vi "Taikoi_GetSystemStatus.vi"(8 "error in (no error)":errorcluster, 10 "LBSysStatRef":refnum<vi>, 11 "USBIdx":i32) -> (0 "error out":errorcluster, 1 "QError":bool, 2 "needUpdate":bool, 3 "Status":string)   [LabVIEW 2019]
uses:
  <userlib>/TaikoLaser/PDLM_Status.ctl
  <userlib>/TaikoLaser/PDLM_NamedBit.ctl
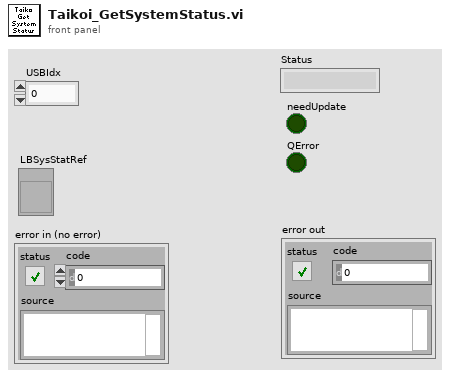
[diagram p1: front panel]
types:
  T1 = typedef "PDLM_Status.ctl" = T2[]
  T2 = typedef "PDLM_NamedBit.ctl" = cluster{"StatName":string, "StatBit":bool}
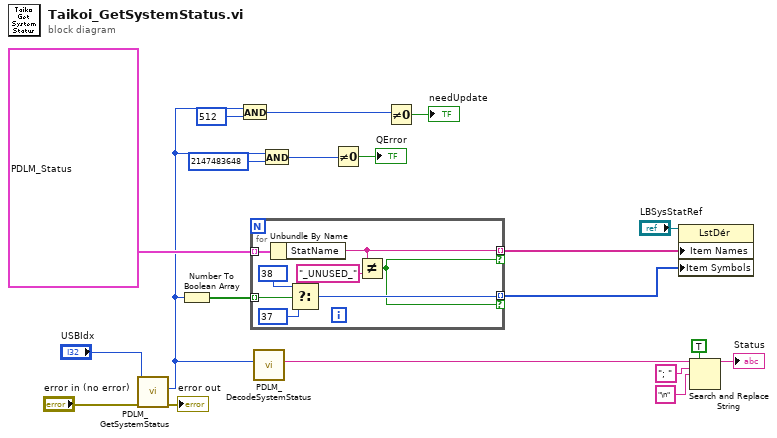
[diagram p0: block diagram]
diagram:
  n1 = call <userlib>:"PDLM_GetSystemStatus.vi"("error in (no error)"="error in (no error)", "USBIdx"="USBIdx") -> ("error out"=→"error out":errorcluster, "state"=w3:u32)  [unwired: 7 in, 1 out]
  n2 = Number To Boolean Array(number=w3) -> (Boolean array=w17:bool[])
  n3 = And(x=w3, y=u32 512) -> (x .and. y?=w6:u32)
  n4 = for {
    tunnel: w17 -> [w27] mode=indexing
    tunnel: T1 [{"StatName"="INITIALIZING", "StatBit"=FALSE}, {"StatName"="DEVICE_UNCALIBRATED", "StatBit"=FALSE}, {"StatName"="COMMISSIONING_MODE", "StatBit"=FALSE}, {"StatName"="LASERHEAD_SAFETY_MODE", "StatBit"=FALSE}, {"StatName"="FW_UPDATE_RUNNING", "StatBit"=FALSE}, {"StatName"="DEVICE_DEFECT", "StatBit"=FALSE}, {"StatName"="DEVICE_INCOMPATIBLE", "StatBit"=FALSE}, {"StatName"="BUSY", "StatBit"=FALSE}, {"StatName"="EXCLUSIVE_SW_OP_GRANTED", "StatBit"=FALSE}, {"StatName"="PARAMETER_CHANGES_PENDING", "StatBit"=FALSE}, {"StatName"="_UNUSED_", "StatBit"=FALSE}, {"StatName"="LASERHEAD_CHANGED", "StatBit"=FALSE}, {"StatName"="LASERHEAD_MISSING", "StatBit"=FALSE}, {"StatName"="LASERHEAD_DEFECT", "StatBit"=FALSE}, {"StatName"="LASERHEAD_UNKNOWN_TYPE", "StatBit"=FALSE}, {"StatName"="LASERHEAD_DECALIBRATED", "StatBit"=FALSE}, {"StatName"="LASERHEAD_DIODE_TEMP_TOO_LOW", "StatBit"=FALSE}, {"StatName"="LASERHEAD_DIODE_TEMP_TOO_HIGH", "StatBit"=FALSE}, {"StatName"="LASERHEAD_DIODE_OVERHEATING", "StatBit"=FALSE}, {"StatName"="LASERHEAD_CASE_OVERHEATING", "StatBit"=FALSE}, {"StatName"="LASERHEAD_FAN_RUNNING", "StatBit"=FALSE}, {"StatName"="LASERHEAD_INCOMPATIBLE", "StatBit"=FALSE}, {"StatName"="LOCKED_BY_EXPIRED_DEMO_MODE", "StatBit"=FALSE}, {"StatName"="LOCKED_BY_ON_OFF_BUTTON", "StatBit"=FALSE}, {"StatName"="SOFTLOCK", "StatBit"=FALSE}, {"StatName"="KEYLOCK", "StatBit"=FALSE}, {"StatName"="LOCKED_BY_SECURITY_POLICY", "StatBit"=FALSE}, {"StatName"="INTERLOCK", "StatBit"=FALSE}, {"StatName"="LASERHEAD_PULSE_POWER_INACCURATE", "StatBit"=FALSE}, {"StatName"="_UNUSED_", "StatBit"=FALSE}, {"StatName"="_UNUSED_", "StatBit"=FALSE}, {"StatName"="ERRORMSG_PENDING", "StatBit"=FALSE}] ("Status") -> [w28] mode=indexing
    tunnel: [w21] -> w18 mode=indexing if=w22
    tunnel: [w24] -> w19 mode=indexing if=w22
    n5 = Unbundle By Name(w28) -> ("StatName"=w21:string)
    n6 = Select(t=38, s=w27, f=37) -> (s? t:f=w24:i32)
    n7 = Not Equal?(x=w21, y="_UNUSED_") -> (x != y?=w22:bool)
  }
  n8 = call <userlib>:"PDLM_DecodeSystemStatus.vi"("state"=w3) -> ("Buffer"=w11:string)  [unwired: 8 in, 2 out]
  n9 = And(x=w3, y=u32 2147483648) -> (x .and. y?=w2:u32)
  n10 = Not Equal To 0?(x=w2) -> (x != 0?=→"QError":bool)
  n11 = Not Equal To 0?(x=w6) -> (x != 0?=→"needUpdate":bool)
  n12 = property class="LstDér"(reference="LBSysStatRef", "Item Names"=w18, "Item Symbols"=w19) -> ()  [unwired: 1 in, 2 out]
  n13 = Search and Replace String(replace all?=TRUE ("replace all? (F)"), input string=w11, search string="; ", replace string="\n" ("replace string (\"\")")) -> (result string=→"Status":string)  [unwired: 4 in, 3 out]
